vi "Is TBS-B Series Model.vi"(8 "error in (no error)":errorcluster, 11 "VISA resource name":refnum<visa-resource-name>) -> (0 "error out":errorcluster, 2 "Is TBS-B Series Model":bool, 3 "VISA resource name out":refnum<visa-resource-name>)   [LabVIEW 2012, in "Tektronix TDS 200 1000 2000 Series.lvlib"]
doc: "Determines whether the current model belongs to TBS-B Series (TBS1052B, TBS1072B, TBS1102B, TBS1152B, TBS1202B)."
uses:
  <instrlib>/Tektronix TDS 200 1000 2000 Series/Tektronix TDS 200 1000 2000 Series.lvlib
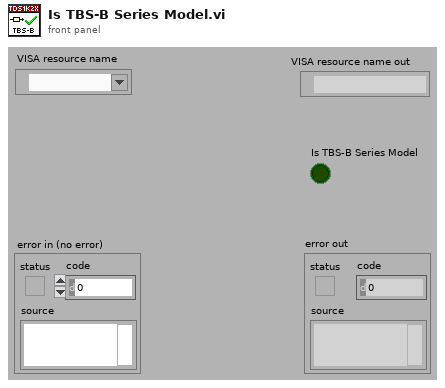
[diagram p1: front panel]
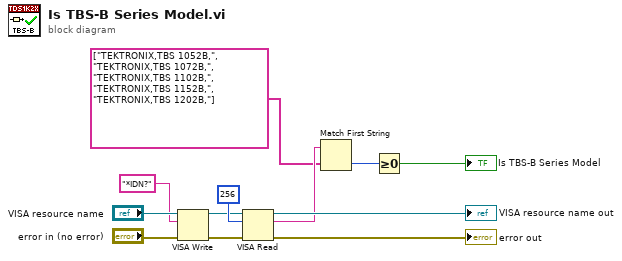
[diagram p0: block diagram]
diagram:
  n1 = VISA Write(VISA resource name="VISA resource name", write buffer="*IDN?", error in (no error)="error in (no error)") -> (VISA resource name out=w8:refnum<visa-resource-name>, error out=w7:errorcluster)  [unwired: 1 out]
  n2 = VISA Read(VISA resource name=w8, byte count=u32 256, error in (no error)=w7) -> (VISA resource name out=→"VISA resource name out":refnum<visa-resource-name>, read buffer=w4:string, error out=→"error out":errorcluster)  [unwired: 1 out]
  n3 = Match First String(2:string[] ["TEKTRONIX,TBS 1052B,", "TEKTRONIX,TBS 1072B,", "TEKTRONIX,TBS 1102B,", "TEKTRONIX,TBS 1152B,", "TEKTRONIX,TBS 1202B,"] ("string array"), 3:w4) -> (0:w2:i32)  [unwired: 1 out]
  n4 = Greater Or Equal To 0?(x=w2) -> (x >= 0?=→"Is TBS-B Series Model":bool)
